vi "Add Buffers.vi"(6 "Decimation":u64, 8 "error in (no error)":errorcluster, 9 "Buffers":refnum<class "Buffers.lvclass">, 10 "parent tag":string, 11 "Application Data In":T1) -> (0 "error out":errorcluster, 3 "Application Data out":T1)   [LabVIEW 2017, in "DSF Data Viewer.lvlib"]
uses:
  DSF Data Viewer.lvlib
  Main VI/Application Data.ctl
  Builds/Data Sharing Framework/Current/Core/DSF Core.lvlibp/Engine/Classes/Framework/Framework.lvclass
  <vilib>/NI/Memory Manager/Classes/Pointer/Pointer.lvclass
  Buffer Reader/Buffer Data.ctl
  Builds/Data Sharing Framework/Current/Core/DSF Core.lvlibp/Engine/Classes/Buffer/Buffer.lvclass
  Builds/Data Sharing Framework/Current/Core/DSF Core.lvlibp/Engine/Classes/Buffer/Buffers.lvclass
  ID to Tree Items/Tree Item Type.ctl
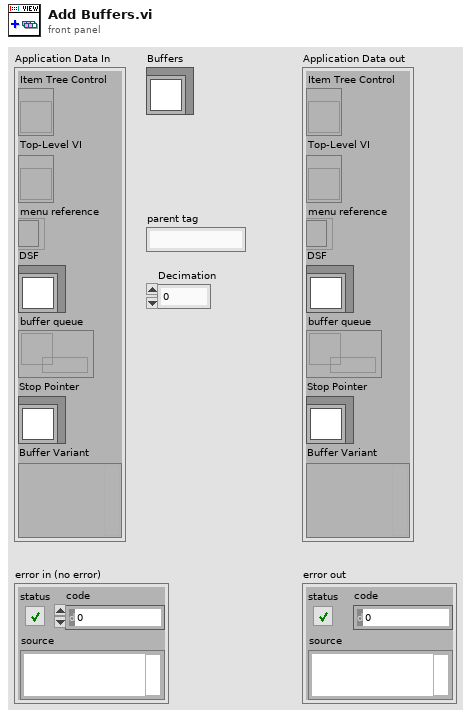
[diagram p1: front panel]
types:
  T1 = typedef "DSF Data Viewer.lvlib/Application Data.ctl" = cluster{"Item Tree Control":refnum<vi>, "Top-Level VI":refnum<vi>, "menu reference":refnum<k9>, "DSF":refnum<class "Framework.lvclass">, "buffer queue":refnum<queue>, "Stop Pointer":refnum<class "Pointer.lvclass">, "Buffer Variant":variant}
  T2 = typedef "DSF Data Viewer.lvlib/Buffer Data.ctl" = cluster{"Buffer":refnum<class "Buffer.lvclass">, "decimation":u64}
  T3 = typedef "DSF Data Viewer.lvlib/Tree Item Type.ctl" = enum16{"Framework", "Plugin Group", "Plugin", "Group", "Transfer", "Buffer", "Channel"}
  T4 = typedef "DSF Data Viewer.lvlib/Tree Item.ctl" = cluster{"Left Cell String":string, "Child Text":string[], "Child Tag":string, "Glyph Index":i32}
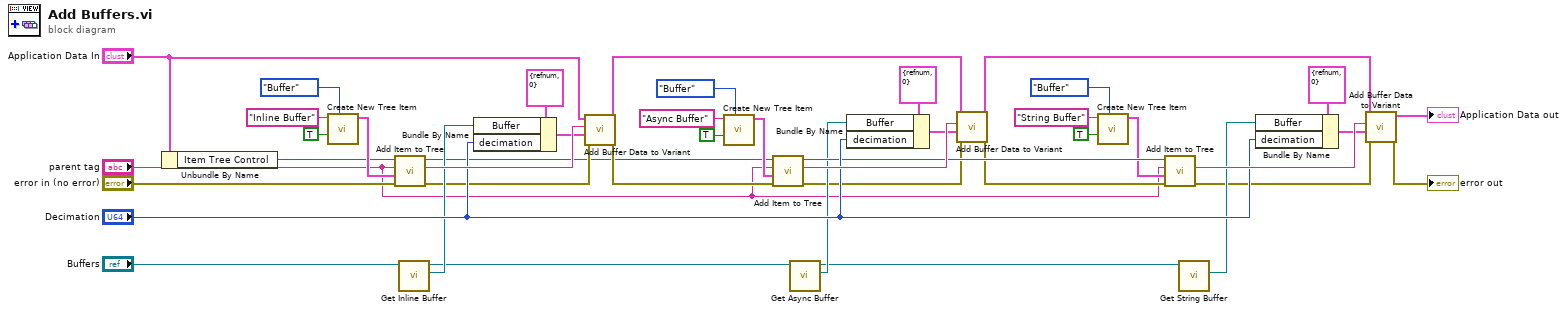
[diagram p0: block diagram]
diagram:
  n1 = Unbundle By Name("Application Data In") -> ("Item Tree Control"=w2:refnum<vi>)
  n2 = call "Create New Tree Item.vi"("Item Type"=Tree_Item_Type."Buffer", "found?"=TRUE, "Left Cell String"="Inline Buffer") -> ("Item"=w5:T4)  [unwired: 7 in, 1 out]
  n3 = call "Add Item to Tree.vi"("error in (no error)"="error in (no error)", "Item"=w5, "parent tag"="parent tag", "TreeControl in"=w2) -> ("error out"=w23:errorcluster, "new item tag"=w41:string, "TreeControl out"=w17:refnum<vi>)  [unwired: 5 in]
  n4 = call "Get Inline Buffer.vi"("Buffers in"="Buffers") -> ("Inline Buffer"=w25:refnum<class "Buffer.lvclass">, "Buffers out"=w12:refnum<class "Buffers.lvclass">)  [unwired: 9 in]
  n5 = Bundle By Name(cluster=T2 {"Buffer"=refnum, "decimation"=0} ("Buffer data"), "Buffer"=w25, "decimation"="Decimation") -> (w22:T2)
  n6 = call "Add Buffer Data to Variant.vi"("error in (no error)"=w23, "Buffer data"=w22, "tag"=w41, "Application Data In in"="Application Data In") -> ("error out"=w24:errorcluster, "Application Data In out"=w28:T1)  [unwired: 6 in]
  n7 = call "Create New Tree Item.vi"("Item Type"=Tree_Item_Type."Buffer", "found?"=TRUE, "Left Cell String"="Async Buffer") -> ("Item"=w18:T4)  [unwired: 7 in, 1 out]
  n8 = call "Add Item to Tree.vi"("error in (no error)"=w24, "Item"=w18, "parent tag"="parent tag", "TreeControl in"=w17) -> ("error out"=w29:errorcluster, "new item tag"=w42:string, "TreeControl out"=w32:refnum<vi>)  [unwired: 5 in]
  n9 = call "Get Async Buffer.vi"("Buffers in"=w12) -> ("Async Buffer"=w31:refnum<class "Buffer.lvclass">, "Buffers out"=w4:refnum<class "Buffers.lvclass">)  [unwired: 9 in]
  n10 = Bundle By Name(cluster=T2 {"Buffer"=refnum, "decimation"=0} ("Buffer data"), "Buffer"=w31, "decimation"="Decimation") -> (w27:T2)
  n11 = call "Add Buffer Data to Variant.vi"("error in (no error)"=w29, "Buffer data"=w27, "tag"=w42, "Application Data In in"=w28) -> ("error out"=w30:errorcluster, "Application Data In out"=w35:T1)  [unwired: 6 in]
  n12 = call "Create New Tree Item.vi"("Item Type"=Tree_Item_Type."Buffer", "found?"=TRUE, "Left Cell String"="String Buffer") -> ("Item"=w19:T4)  [unwired: 7 in, 1 out]
  n13 = call "Add Item to Tree.vi"("error in (no error)"=w30, "Item"=w19, "parent tag"="parent tag", "TreeControl in"=w32) -> ("error out"=w37:errorcluster, "new item tag"=w43:string)  [unwired: 5 in, 1 out]
  n14 = call "Get String Buffer.vi"("Buffers in"=w4) -> ("String Buffer"=w39:refnum<class "Buffer.lvclass">)  [unwired: 9 in, 1 out]
  n15 = Bundle By Name(cluster=T2 {"Buffer"=refnum, "decimation"=0} ("Buffer data"), "Buffer"=w39, "decimation"="Decimation") -> (w34:T2)
  n16 = call "Add Buffer Data to Variant.vi"("error in (no error)"=w37, "Buffer data"=w34, "tag"=w43, "Application Data In in"=w35) -> ("error out"=→"error out":errorcluster, "Application Data In out"=→"Application Data out":T1)  [unwired: 6 in]
